vi "Manual Scale.vi"(8 "error in (no error)":errorcluster, 9 "Secs/div":dbl, 10 "V/div":T1, 11 "MSOX6004 in":refnum<class "MSOX6004.lvclass">) -> (0 "error out":errorcluster, 3 "MSOX6004 out":refnum<class "MSOX6004.lvclass">)   [LabVIEW 2018, in "MSOX6004.lvlib" / "MSOX6004.lvclass"]
doc: "This Overrride is used to manually adjust the scale of the instrument."
uses:
  MSOX6004.lvclass
  PPLs/Oscilloscope/Parent/Oscilloscope.lvlibp/Custom Controls/Volts per Division.ctl
  PPLs/Oscilloscope/Parent/Oscilloscope.lvlibp/Custom Controls/Analog Channels.ctl
  MSOX6004.lvclass/MSOX6004.ctl
  <instrlib>/Keysight InfiniiVision/Keysight InfiniiVision.lvlib
  PPLs/Oscilloscope/Parent/Oscilloscope.lvlibp
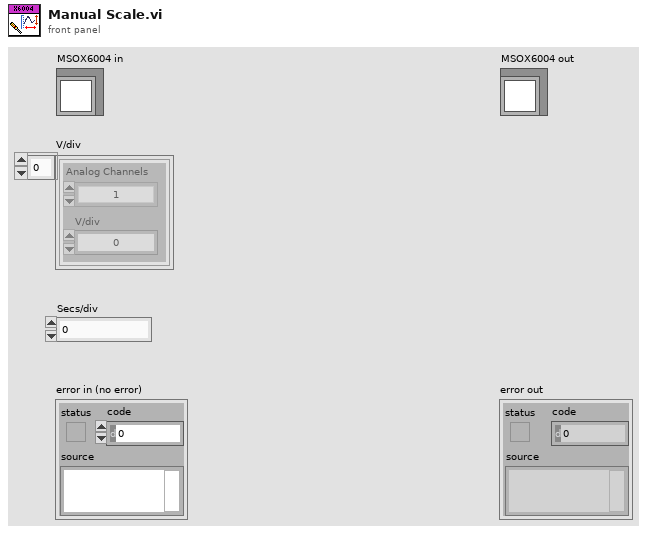
[diagram p1: front panel]
types:
  T1 = typedef "Oscilloscope.lvlibp/Volts per Division.ctl" = cluster{"Analog Channels":T2, "V/div":dbl}[]
  T2 = typedef "Oscilloscope.lvlibp/Analog Channels.ctl" = enum16{"1", "2", "3", "4", "5", "6", "7", "8", "9", "10", "11", "12", "13", "14", "15", "16"}
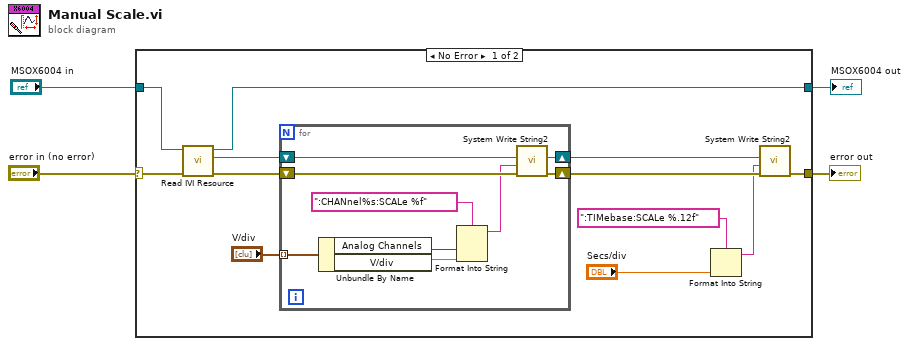
[diagram p0: block diagram]
diagram:
  n1 = case shown="No Error" "error in (no error)" {
    selector: "error in (no error)" -> [w16 w27]
    tunnel: [w5 w27] -> w3
    tunnel: [w12 w26] -> w2
    tunnel: "MSOX6004 in" -> [w15 w26]
    frame No Error {
      n2 = call "Read IVI Resource.vi"("error in (no error)"=w16, "MSOX6004 in"=w15) -> ("error out"=w13:errorcluster, "IVI Resource"=w11:refnum<k15>, "MSOX6004 out"=w12:refnum<class "MSOX6004.lvclass">)  [unwired: 7 in]
      n3 = for {
        tunnel: "V/div" -> [w25] mode=indexing
        shift-right: [w23] -> w8
        shift-left: w13 -> [w24]
        shift-right: [w17] -> w7
        shift-left: w11 -> [w22]
        n4 = Unbundle By Name(w25) -> ("Analog Channels"=w20:T2, "V/div"=w19:dbl)
        n5 = Format Into String(format string=":CHANnel%s:SCALe %f", w20, w19) -> (resulting string=w18:string)  [unwired: 2 in, 1 out]
        n6 = call <instrlib>:"System Write String2.vi"("error in (no error)"=w24, "Data"=w18, "instrument handle"=w22) -> ("error out"=w23:errorcluster, "instrument handle out"=w17:refnum<k15>)  [unwired: 7 in]
      }
      n7 = Format Into String(format string=":TIMebase:SCALe %.12f", "Secs/div") -> (resulting string=w6:string)  [unwired: 2 in, 1 out]
      n8 = call <instrlib>:"System Write String2.vi"("error in (no error)"=w8, "Data"=w6, "instrument handle"=w7) -> ("error out"=w5:errorcluster)  [unwired: 7 in, 1 out]
    }
    frame Error {
    }
  }
  "error out" <- w3
  "MSOX6004 out" <- w2
